vi "prg_inp.vi"(6 "options":i32=128 format="%.0x", 7 "Reset to default":bool, 8 "error in (no error)":errorcluster, 9 "Name":string, 10 "machine name (\"\":  open local reference)":string, 11 "vi path":path) -> (0 "error out":errorcluster)   [LabVIEW 2015]
doc: "Set the reaction VI that will be called when a tuple with \"name\" in read from tuple space."
uses:
  C:/Users/Giuseppe/Downloads/LabLinda_ pakage/index_datatype.ctl
  C:/Users/Giuseppe/Downloads/LabLinda_ pakage/index_cluster.ctl
panel:
  in  "Options":i32=64 format="%x"
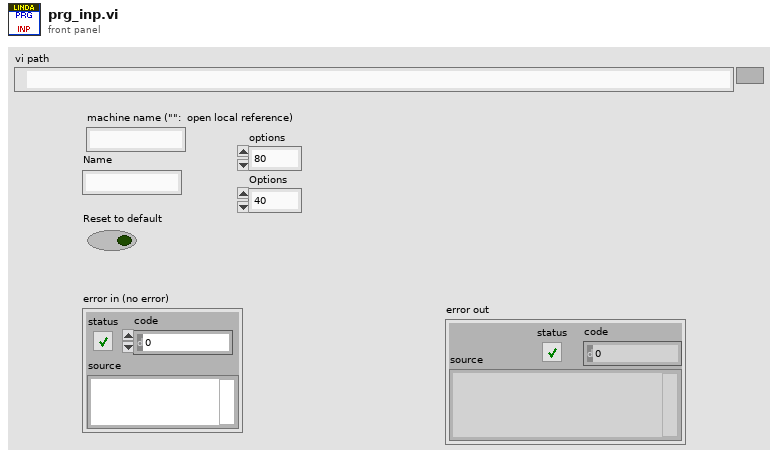
[diagram p1: front panel]
types:
  T1 = typedef "index_datatype.ctl" = T2[]
  T2 = typedef "index_cluster.ctl" = cluster{"Addr":i32[], "out react vi reference":refnum<vi>, "in react vi reference":refnum<vi>, "rd react vi reference":refnum<vi>, "Read_write_var":refnum<vi>}
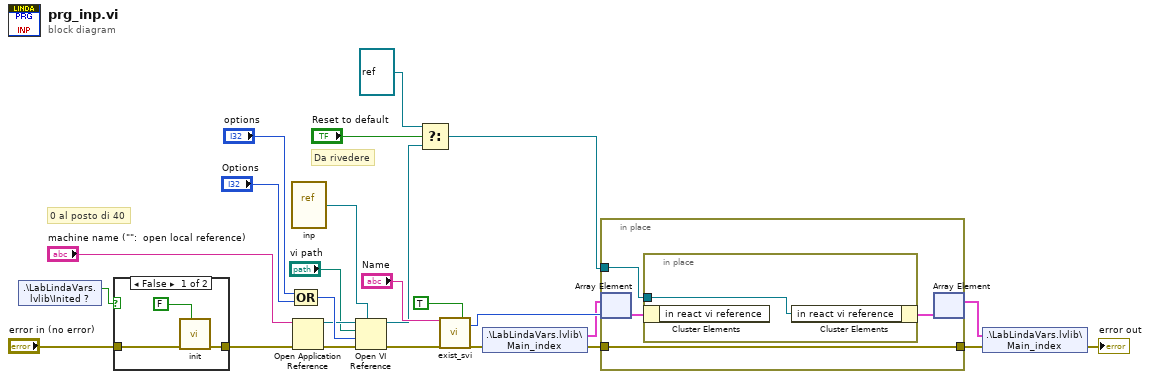
[diagram p0: block diagram]
diagram:
  # "Da rivedere"
  # "0 al posto di 40"
  n1 = shared-variable ".\\LabLindaVars.lvlib\\Inited ?"() -> (w9:bool)  [unwired: 1 in, 1 out]
  n2 = case shown="False" w9 {
    tunnel: [w28 w29] -> w7
    tunnel: "error in (no error)" -> [w27 w29]
    frame False {
      n3 = call "init.vi"("Cleaneup"=FALSE ("Cleneup"), "error in (no error)"=w27) -> ("error out"=w28:errorcluster)  [unwired: 9 in]
    }
    frame True {
    }
  }
  n4 = vi-ref "inp.vi"() -> (w6:refnum<vi>)
  n5 = Open Application Reference(8:w7, 11:"machine name (\"\":  open local reference)") -> (0:w13:errorcluster, 3:w11:refnum<vi>)  [unwired: 2 in]
  n6 = Compound Arithmetic op=OR("options", "Options") -> (w23:i32)
  n7 = Open VI Reference(type specifier VI Refnum (for type only)=w6, application reference (local)=w11, vi path="vi path", options=w23, error in (no error)=w13) -> (vi reference=w5:refnum<vi>, error out=w10:errorcluster)  [unwired: 1 in]
  n8 = Select(t=refnum<vi> refnum, s="Reset to default", f=w5) -> (s? t:f=w4:refnum<vi>)
  n9 = call "exist_svi.vi"("Name"="Name", "error in (no error)"=w10, "Create ?"=TRUE) -> ("index of element"=w20:i32, "error out"=w17:errorcluster)  [unwired: 13 in, 2 out]
  n10 = shared-variable ".\\LabLindaVars.lvlib\\Main_index"(error in=w17) -> (w18:T1, error out=w16:errorcluster)
  n11 = in-place {
    in-place-border: w4 -> [w31]
    in-place-border: [w30] -> w15
    in-place-border: w16 -> [w30]
    n12 = in-place-array #1(w18, w20) -> (w33:T2)
    n13 = in-place {
      in-place-border: w31 -> [w34]
      n14 = in-place-cluster #2(w33) -> ()  [unwired: 1 out]
      n15 = in-place-cluster #2("in react vi reference"=w34) -> (w32:T2)
    }
    n16 = in-place-array #1(w32) -> (w19:T1)  [unwired: 1 out]
  }
  n17 = shared-variable ".\\LabLindaVars.lvlib\\Main_index"(w19, error in=w15) -> (error out=→"error out":errorcluster)
